vi "getOutputVoltage.vi"(8 "error in":errorcluster, 10 "axis in":u8, 11 "connection ID":refnum<k5>) -> (0 "error out":errorcluster, 1 "Voltage (mv)":i64, 2 "axis out":u8, 3 "connection ID":refnum<k5>)   [LabVIEW 2019]
panel:
  in  "Get Command":string="com.attocube.amc.control.getCurrentOutputVoltage"
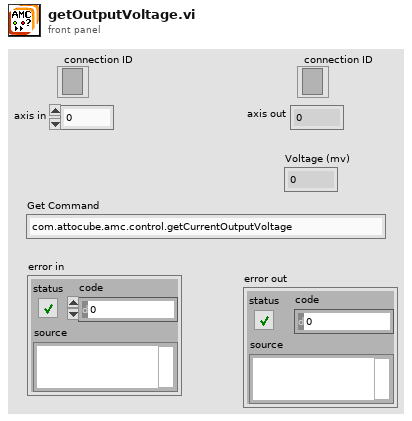
[diagram p1: front panel]
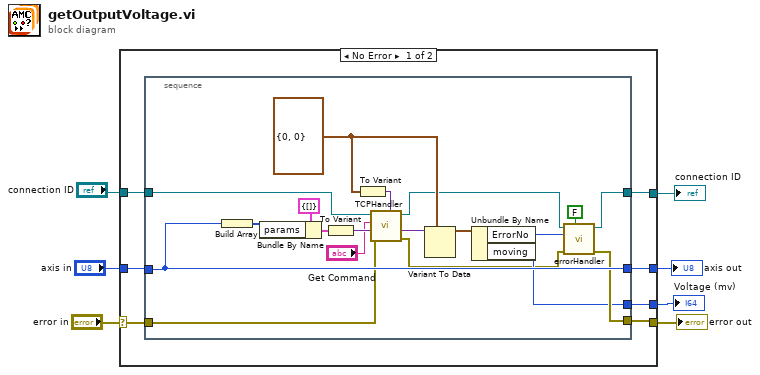
[diagram p0: block diagram]
diagram:
  n1 = case shown="No Error" "error in" {
    selector: "error in" -> [w8 w35]
    tunnel: "axis in" -> [w14 w36]
    tunnel: [w10 w35] -> w6
    tunnel: [w11 w36] -> w5
    tunnel: [w12 w34] -> w4
    tunnel: "connection ID" -> [w13 w34]
    tunnel: [w9 _] -> w1
    frame No Error {
      n2 = stacked-sequence {
        tunnel: [w19] -> w12
        tunnel: w13 -> [w23]
        tunnel: w14 -> [w25]
        tunnel: [w25] -> w11
        tunnel: [w24] -> w10
        tunnel: [w18] -> w9
        tunnel: w8 -> [w16]
        frame #0 {
          w21 = cluster{"ErrorNo":i32, "moving":i64} {"ErrorNo"=0, "moving"=0} ("input cluster")
          n3 = Build Array(w25) -> (w29:u8[])
          n4 = Bundle By Name(cluster=cluster{"params":i32[]} {"params"=[]} ("input cluster"), "params"=w29) -> (w30:cluster{"params":i32[]})
          n5 = To Variant(anything=w30) -> (Variant=w31:variant)
          n6 = To Variant(anything=w21) -> (Variant=w22:variant)
          n7 = call <userlib>:"TCPHandler.vi"("result Types"=w22, "error in (no error)"=w16, "params"=w31, "method"="Get Command", "connection ID"=w23) -> ("error out"=w15:errorcluster, "result"=w27:variant, "connection ID"=w20:refnum<k5>)  [unwired: 3 in, 1 out]
          n8 = Variant To Data(type=w21, Variant=w27) -> (data=w32:cluster{"ErrorNo":i32, "moving":i64})  [unwired: 1 in, 1 out]
          n9 = Unbundle By Name(w32) -> ("ErrorNo"=w33:i32, "moving"=w18:i64)
          n10 = call <userlib>:"errorHandler.vi"("show popup"=FALSE, "error in"=w15, "error number"=w33, "connection ID"=w20) -> ("error out"=w24:errorcluster, "connection ID"=w19:refnum<k5>)  [unwired: 6 in]
        }
      }
    }
    frame Error {
    }
  }
  "error out" <- w6
  "axis out" <- w5
  "connection ID" <- w4
  "Voltage (mv)" <- w1
